vi "Convert IMAQ to OpenCV.vi"() -> ()   [LabVIEW 2017]
uses:
  IMAQCV/IMAQCV.lvlib
panel:
  out "Display Picture":picture
  out "error out":errorcluster
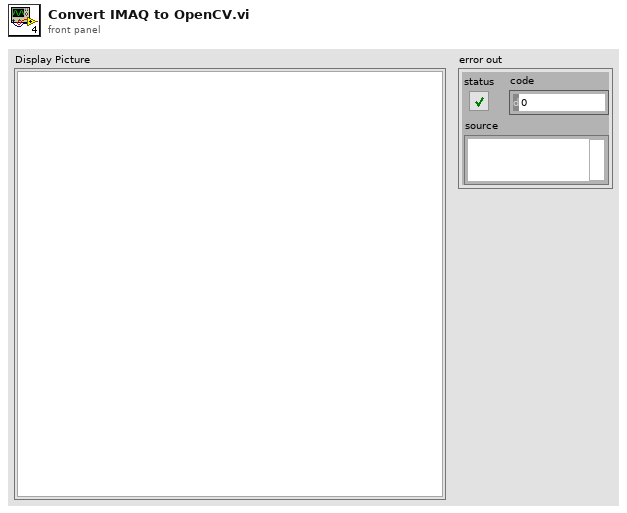
[diagram p1: front panel]
types:
  T1 = typedef "Image Type" = u32
  T2 = typedef "IMAQCV.lvlib/IMAQCV Image.ctl" = refnum<vi>
  T3 = typedef "IMAQ Image.ctl" = refnum<image>
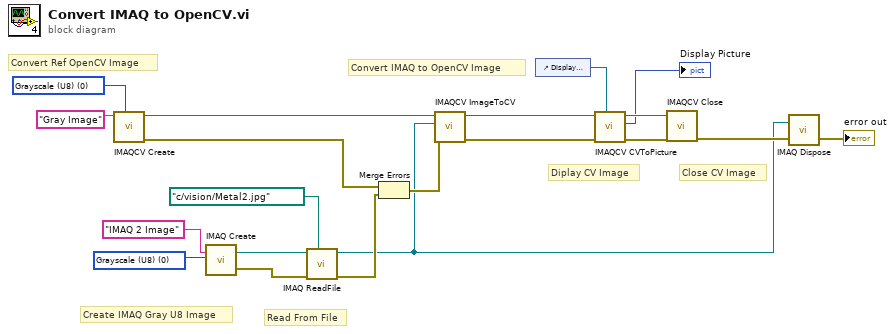
[diagram p0: block diagram]
diagram:
  w16 = T1 0 items=["Grayscale (U8)", "Grayscale (I16)", "Grayscale (SGL)", "Complex (CSG)", "RGB (U32)", "HSL (U32)", "RGB (U64)", "Grayscale (U16)"] ("Image Type")
  w6 = u32 0 items=["Grayscale (U8)", "Grayscale (I16)", "Grayscale (SGL)", "Complex (CSG)", "RGB (U32)", "HSL (U32)", "RGB (U64)", "Grayscale (U16)"] ("Image Type")
  # "Convert Ref OpenCV Image"
  # "Convert IMAQ to OpenCV Image"
  # "Close CV Image"
  # "Diplay CV Image"
  # "Read From File"
  # "Create IMAQ Gray U8 Image"
  n1 = call "IMAQCV Create.vi"("Image Type"=w6, "Image Name"="Gray Image") -> ("error out"=w11:errorcluster, "Image Out"=w14:T2)  [unwired: 8 in]
  n2 = call "IMAQ Create"("Image Name"="IMAQ 2 Image", "Image Type"=w16) -> ("New Image"=w18:T3, "error out"=w17:errorcluster)  [unwired: 2 in, 1 out]
  n3 = call "IMAQ ReadFile"("File Path"=path "c:/vision/Metal2.jpg" ("appended path"), "error in (no error)"=w17, "Image"=w18) -> ("error out"=w12:errorcluster, "Image Out"=w2:T3)  [unwired: 2 in, 5 out]
  n4 = Merge Errors(w11, w12) -> (w13:errorcluster)
  n5 = call "IMAQCV ImageToCV.vi"("error in (no error)"=w13, "Variant In"=w2, "CV in"=w14) -> ("error out"=w10:errorcluster, "CV out"=w9:T2)  [unwired: 7 in]
  n6 = control-ref of="Display Picture"() -> (w1:refnum<vi>)
  n7 = call "IMAQCV CVToPicture.vi"("picture ref"=w1, "error in (no error)"=w10, "image"=w9) -> ("error out"=w8:errorcluster, "picture"=→"Display Picture":picture, "image out"=w7:T2)  [unwired: 6 in]
  n8 = call "IMAQCV Close.vi"("error in (no error)"=w8, "Image"=w7) -> ("error out"=w4:errorcluster)  [unwired: 9 in]
  n9 = call "IMAQ Dispose"("Image"=w2, "error in (no error)"=w4) -> ("error out"=→"error out":errorcluster)  [unwired: 4 in]
